vi "Read Result.vi"(8 "error in (no error)":errorcluster, 11 "Measurement path":path) -> (0 "error out":errorcluster, 2 "Result (val, unc)":string[][](array[string]))   [LabVIEW 2020]
uses:
  external libraries/TWM-1.8.7.0-client/Get 2D EXT.vi
  external libraries/TWM-1.8.7.0-client/infolib.lvlib
panel:
  out "rms section exist":bool
  out "u1 section exist":bool
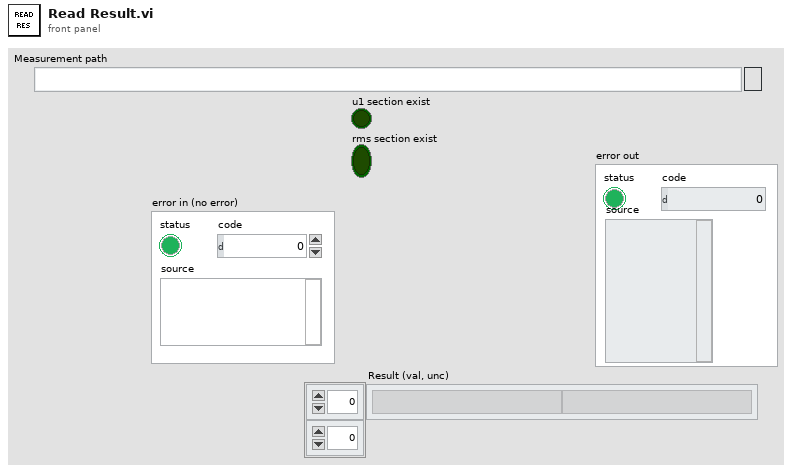
[diagram p1: front panel]
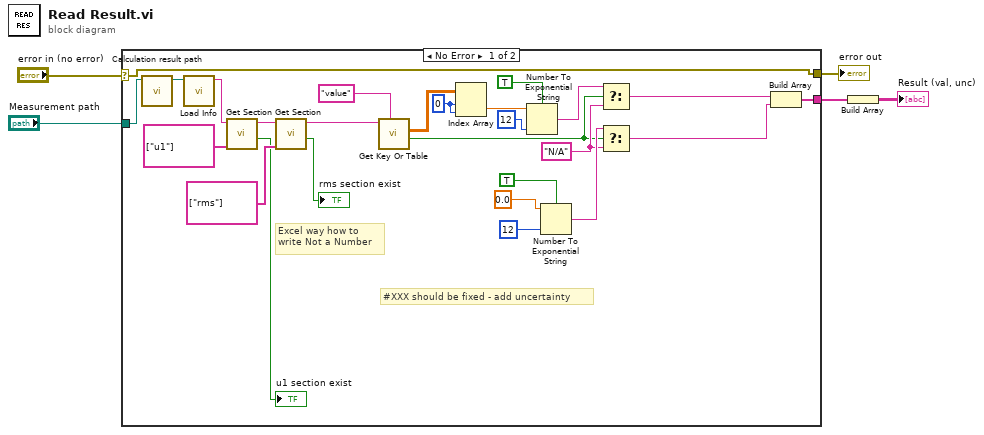
[diagram p0: block diagram]
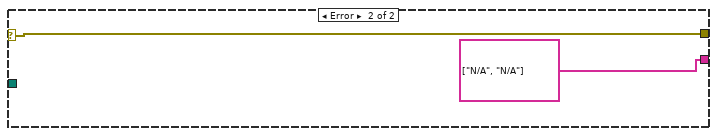
[diagram p2: hidden frame]
diagram:
  n1 = case shown="No Error" "error in (no error)" {
    selector: "error in (no error)" -> [w31 w33]
    tunnel: [w31 w33] -> w4
    tunnel: [w26 string[] ["N/A", "N/A"]] -> w3
    tunnel: "Measurement path" -> [w24 _]
    frame No Error {
      w14 = 0 ("index (row)")
      w20 = "N/A" ("f")
      # "#XXX should be fixed - add uncertainty"
      # "Excel way how to\nwrite Not a Number"
      n2 = call "Calculation result path.vi"("Measurement path"=w24) -> ("calc result info path"=w10:path)  [unwired: 9 in, 1 out]
      n3 = call "Load Info.vi"("filename"=w10) -> ("info data"=w18:string)  [unwired: 9 in, 1 out]
      n4 = call "Get Section.vi"("sections"=string[] ["u1"], "info data"=w18) -> ("exist"=→"u1 section exist":bool, "section part"=w17:string)  [unwired: 7 in, 1 out]
      n5 = call "Get Section.vi"("sections"=string[] ["rms"], "info data"=w17) -> ("exist"=→"rms section exist":bool, "section part"=w16:string)  [unwired: 7 in, 1 out]
      n6 = call-poly "Get Key Or Table.vi"("key description"="value", "info data"=w16) -> ("key found?"=w8:bool, "value"=w15:ext[][])  [unwired: 6 in, 2 out]
      n7 = Index Array(array=w15, index (row)=w14, index (col)=w14) -> (element=w9:ext)
      n8 = Number To Exponential String(number=w9, precision (6)=i16 12, 1:TRUE ("use system decimal point (T)")) -> (E-format string=w21:string)  [unwired: 1 in]
      n9 = Number To Exponential String(number=0.0, precision (6)=i16 12, 1:TRUE ("use system decimal point (T)")) -> (E-format string=w23:string)  [unwired: 1 in]
      n10 = Select(t=w21, s=w8, f=w20) -> (s? t:f=w19:string)
      n11 = Select(t=w23, s=w8, f=w20) -> (s? t:f=w22:string)
      n12 = Build Array(w19, w22) -> (w26:string[])
    }
    frame Error {
    }
  }
  "error out" <- w4
  n13 = Build Array(w3) -> (→"Result (val, unc)":string[][])
